vi "Counter - Read Encoder Velocity2 (Continuous Clock).vi"() -> ()   [LabVIEW 2015]
doc: "This example demonstrates how to use a counter input along with an external clock to continually sample the angular velocity measured from an encoder.\n\nFor instructions on how to connect your signals to the DAQ device, refer to your device documentation."
uses:
  <vilib>/Utility/error.llb/DialogType.ctl
  <vilib>/DAQmx/read.llb/DAQmx Read (Analog 1D Wfm NChan NSamp).vi
  <vilib>/DAQmx/read.llb/DAQmx Read (Counter 2D DBL NChan NSamp).vi
  <vilib>/DAQmx/create/channels.llb/DAQmx Create Channel (CI-Velocity-Linear).vi
  <vilib>/DAQmx/configure/timing.llb/DAQmx Timing (Sample Clock).vi
  <vilib>/DAQmx/create/channels.llb/DAQmx Create Channel (AI-Voltage-Basic).vi
  <vilib>/DAQmx/miscellaneous.llb/DAQmx Fill In Error Info.vi
  <resource>/objmgr/daqmx.rc
panel:
  out "Stop2":bool
  out "Waveform Chart":dbl(graph)
  out "x-y":u32
  out "Gauge":dbl(knob) scale=0.0..10.0
  in  "Counter 0":tag="Mantis1_1Mod4/ctr0"
  in  "B Input Terminal":tag="/Mantis1_1Mod4/PFI7"
  in  "A Input Terminal":tag="/Mantis1_1Mod4/PFI0"
  in  "Stop":bool
  in  "Samples per Loop":i32=100
  in  "Sample Rate":dbl=1000.0
  in  "Sample Clock Source":tag="OnboardClock"
  # "MPH"
  # "Channel Settings"
  # "Timing Settings"
  # "Trigger Settings"
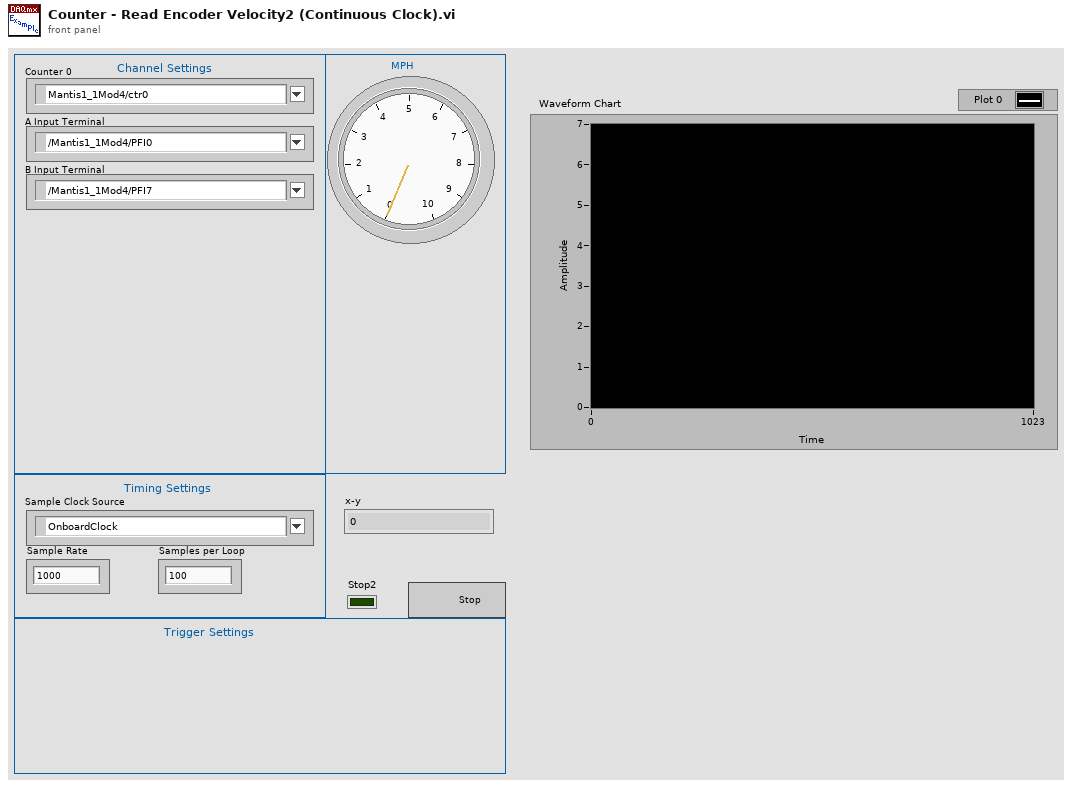
[diagram p1: front panel]
types:
  T1 = typedef "DialogType.ctl" = u16
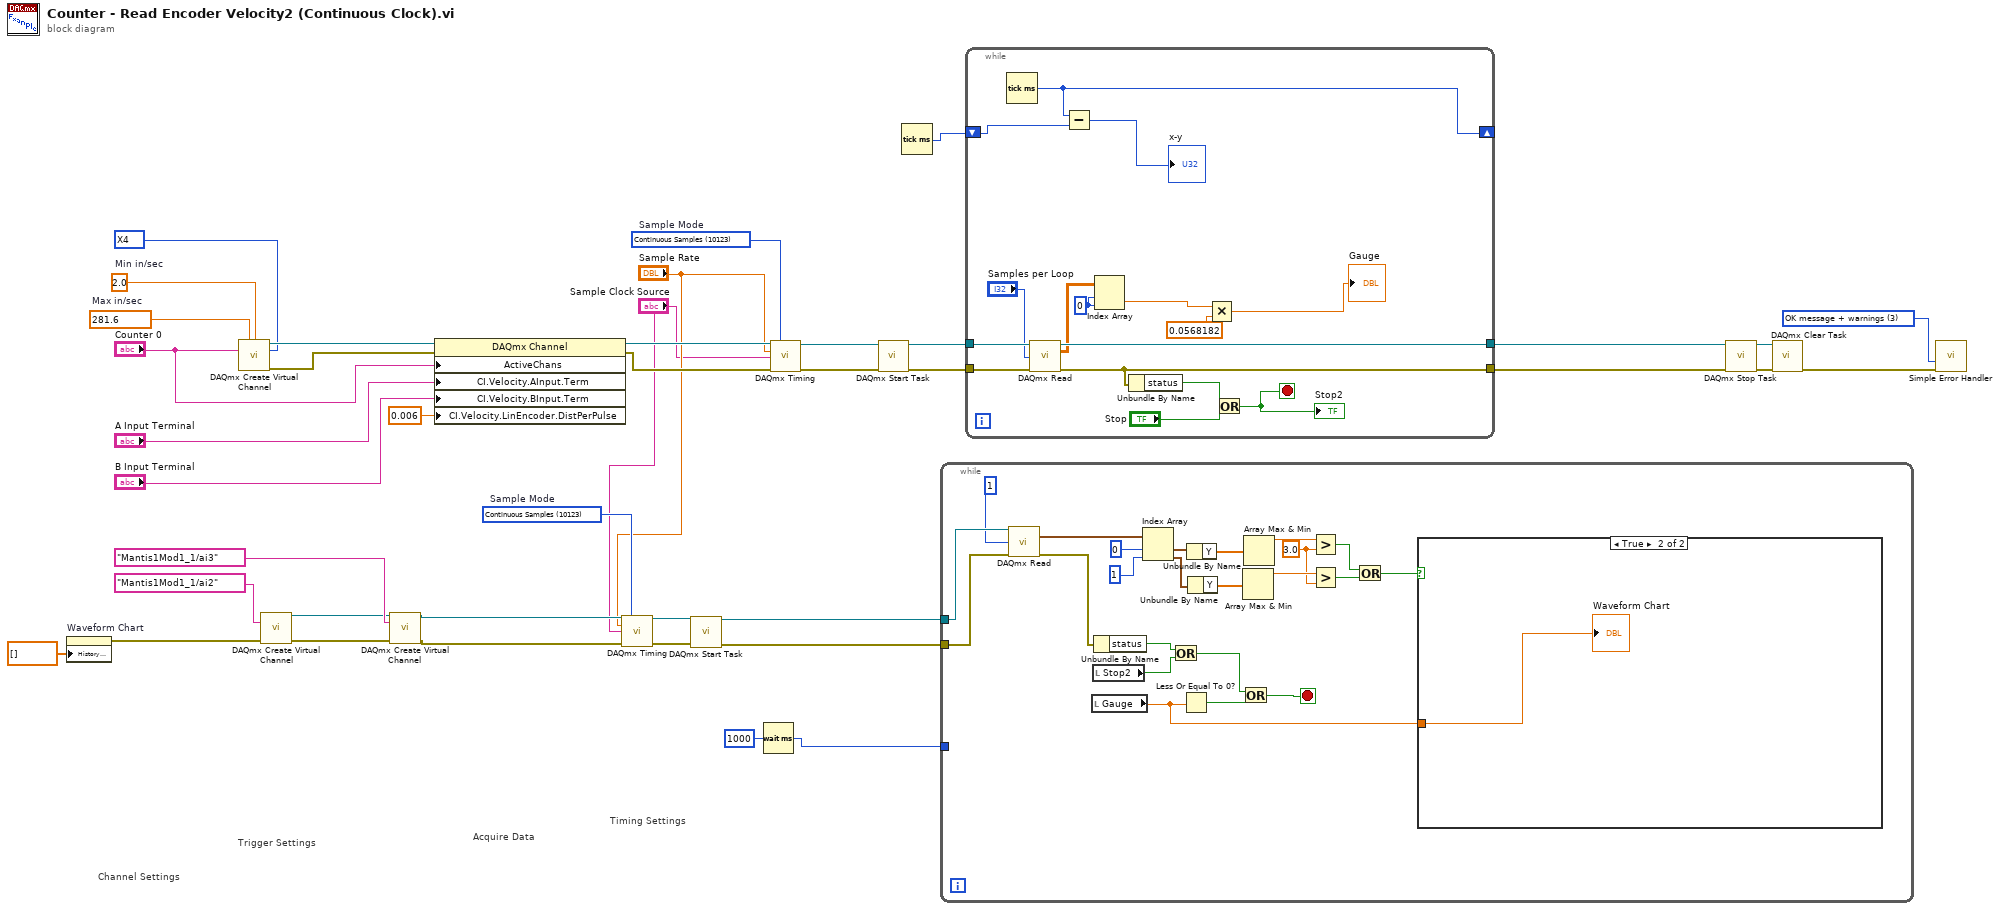
[diagram p0: block diagram]
diagram:
  w13 = 10123 items=["Finite Samples"=10178, "Continuous Samples"=10123, "Hardware Timed Single Point"=12522]  # Sample Mode
  w29 = 281.6  # Max in/sec
  w28 = 2.0  # Min in/sec
  w23 = 10092 items=["X1"=10090, "X2"=10091, "X4"=10092, "Two Pulse Counting"=10313] ("decoding type")
  w32 = T1 3 items=["no dialog", "OK message", "continue or stop message", "OK message + warnings", "continue/stop + warnings"] ("type of dialog (OK msg:1)")
  w40 = 10123 items=["Finite Samples"=10178, "Continuous Samples"=10123, "Hardware Timed Single Point"=12522]  # Sample Mode
  # "Acquire Data"
  # "Trigger Settings"
  # "Timing Settings"
  # "Channel Settings"
  n1 = property on="Waveform Chart" class="WFChart (strict)"("History Data"=dbl[] []) -> (error out=w4:errorcluster)  [unwired: 2 in, 1 out]
  n2 = call-poly <vilib>:"DAQmx Create Virtual Channel.vi"("maximum value"=w29, "minimum value"=w28, "counter"="Counter 0", "decoding type"=w23) -> ("task out"=w31:refnum<k21>, "error out"=w30:errorcluster)  [unwired: 10 in]
  n3 = call-poly <vilib>:"DAQmx Create Virtual Channel.vi"("physical channels"=tag "Mantis1Mod1_1/ai2", "error in"=w4) -> ("task out"=w20:refnum<k21>, "error out"=w19:errorcluster)  [unwired: 12 in]
  n4 = call-poly <vilib>:"DAQmx Create Virtual Channel.vi"("task in"=w20, "physical channels"=tag "Mantis1Mod1_1/ai3", "error in"=w19) -> ("task out"=w12:refnum<k21>, "error out"=w11:errorcluster)  [unwired: 11 in]
  n5 = property class="DAQmx Channel"(reference=w31, error in=w30, "ActiveChans"="Counter 0", "CI.Velocity.AInput.Term"="A Input Terminal", "CI.Velocity.BInput.Term"="B Input Terminal", "CI.Velocity.LinEncoder.DistPerPulse"=0.006) -> (reference out=w17:refnum<k21>, error out=w18:errorcluster)
  n6 = call-poly <vilib>:"DAQmx Timing.vi"("task/channels in"=w12, "sample mode"=w13, "rate"="Sample Rate", "source"="Sample Clock Source", "error in"=w11) -> ("task out"=w8:refnum<k21>, "error out"=w7:errorcluster)  [unwired: 9 in]
  n7 = call <vilib>:"DAQmx Start Task.vi"("task/channels in"=w8, "error in"=w7) -> ("task out"=w6:refnum<k21>, "error out"=w5:errorcluster)  [unwired: 12 in]
  n8 = Wait (ms)(milliseconds to wait=u32 1000) -> (millisecond timer value=w1:u32)
  n9 = call-poly <vilib>:"DAQmx Timing.vi"("task/channels in"=w17, "sample mode"=w40, "rate"="Sample Rate", "source"="Sample Clock Source", "error in"=w18) -> ("task out"=w15:refnum<k21>, "error out"=w16:errorcluster)  [unwired: 9 in]
  n10 = call <vilib>:"DAQmx Start Task.vi"("task/channels in"=w15, "error in"=w16) -> ("task out"=w39:refnum<k21>, "error out"=w38:errorcluster)  [unwired: 12 in]
  n11 = Tick Count (ms)() -> (millisecond timer value=w14:u32)
  n12 = while {
    tunnel: w6 -> [w63]
    tunnel: w5 -> [w62]
    tunnel: w1 -> [_]
    stop <- w42 stop-if-true
    w52 = 3.0 ("y")
    n13 = call-poly <vilib>:"DAQmx Read.vi"("task/channels in"=w63, "number of samples per channel"=1, "error in"=w62) -> ("data"=w49:waveform(dbl)[], "error out"=w48:errorcluster)  [unwired: 10 in, 1 out]
    n14 = local read "Gauge"() -> (w41:dbl)
    n15 = local read "Stop2"() -> (w46:bool)
    n16 = Unbundle By Name(w48) -> ("status"=w47:bool)
    n17 = Index Array(array=w49, index #1=0 ("index"), index #2=1 ("index")) -> (element #1=w59:waveform(dbl), element #2=w56:waveform(dbl))
    n18 = Or(x=w47, y=w46) -> (x .or. y?=w44:bool)
    n19 = Less Or Equal To 0?(x=w41) -> (x <= 0?=w43:bool)
    n20 = Unbundle By Name(w59) -> ("Y"=w58:dbl[])
    n21 = Unbundle By Name(w56) -> ("Y"=w55:dbl[])
    n22 = Or(x=w44, y=w43) -> (x .or. y?=w42:bool)
    n23 = Array Max & Min(array=w55) -> (max value=w53:dbl)  [unwired: 3 out]
    n24 = Array Max & Min(array=w58) -> (max value=w54:dbl)  [unwired: 3 out]
    n25 = Greater?(x=w54, y=w52) -> (0:w51:bool)
    n26 = Greater?(x=w53, y=w52) -> (0:w50:bool)
    n27 = Or(x=w51, y=w50) -> (x .or. y?=w45:bool)
    n28 = case shown="True" w45 {
      tunnel: w41 -> [_ w64]
      frame False {
      }
      frame True {
        "Waveform Chart" <- w64
      }
    }
  }
  n29 = while {
    tunnel: w39 -> [w80]
    tunnel: w38 -> [w79]
    tunnel: [w77] -> w35
    tunnel: [w78] -> w36
    shift-right: [w67] -> _
    shift-left: w14 -> [w68]
    stop <- w65 stop-if-true
    w69 = 0 ("disabled index (col)")
    n30 = Tick Count (ms)() -> (millisecond timer value=w67:u32)
    n31 = call-poly <vilib>:"DAQmx Read.vi"("task/channels in"=w80, "number of samples per channel"="Samples per Loop", "error in"=w79) -> ("task out"=w78:refnum<k21>, "data"=w73:dbl[][], "error out"=w77:errorcluster)  [unwired: 10 in]
    n32 = Subtract(x=w67, y=w68) -> (x-y=→"x-y":u32)
    n33 = Index Array(array=w73, index (row)=w69, index (col)=w69) -> (element=w71:dbl)
    n34 = Unbundle By Name(w77) -> ("status"=w76:bool)
    n35 = Multiply(x=w71, y=0.0568182) -> (x*y=→"Gauge":dbl)
    n36 = Or(x=w76, y="Stop") -> (x .or. y?=w65:bool)
    "Stop2" <- w65
  }
  n37 = call <vilib>:"DAQmx Stop Task.vi"("task/channels in"=w36, "error in"=w35) -> ("task out"=w33:refnum<k21>, "error out"=w34:errorcluster)  [unwired: 12 in]
  n38 = call <vilib>:"DAQmx Clear Task.vi"("task in"=w33, "error in"=w34) -> ("error out"=w37:errorcluster)  [unwired: 13 in]
  n39 = call <vilib>:"Simple Error Handler.vi"("type of dialog (OK msg:1)"=w32, "error in (no error)"=w37) -> ()  [unwired: 3 in, 5 out]
